vi "Blop.vi"(6 "Rec":bool, 8 "Sample In":fxp<+/-,8,8>) -> (0 "Sample Out":fxp<+/-,8,8>)   [LabVIEW 2015]
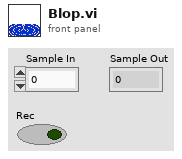
[diagram p1: front panel]
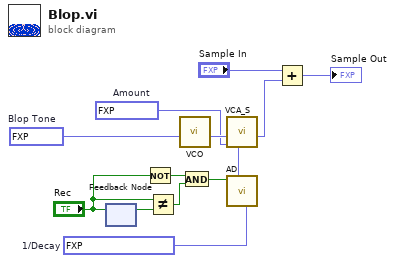
[diagram p0: block diagram]
diagram:
  w6 = fxp<+,32,32> 28091770.0  # Blop Tone
  w4 = fxp<+,8,0> 0.99609375  # Amount
  w2 = fxp<+,16,0> 0.0003814697265625  # 1/Decay
  n1 = feedback #1() -> (w10:bool)  [unwired: 1 in]
  n2 = feedback-in #1("Rec") -> ()
  n3 = Not(x="Rec") -> (.not. x?=w8:bool)
  n4 = Not Equal?(x="Rec", y=w10) -> (x != y?=w7:bool)
  n5 = call "VCO.vi"("M"=w6) -> ("Sine Sample"=w5:fxp<+/-,8,8>)  [unwired: 10 in]
  n6 = And(x=w8, y=w7) -> (x .and. y?=w3:bool)
  n7 = call "AD.vi"("1/Decay"=w2, "Trigger"=w3) -> ("Sample Out"=w1:fxp<+,8,0>)  [unwired: 9 in]
  n8 = call "VCA_S.vi"("EG"=w1, "Amount"=w4, "Sample In"=w5) -> ("Sample Out"=w12:fxp<+/-,8,8>)  [unwired: 8 in]
  n9 = Add(x="Sample In", y=w12) -> (x+y=→"Sample Out":fxp<+/-,8,8>)
